vi "Pulse Generator Trigger.vi"() -> ()   [LabVIEW 2020]
uses:
  <vilib>/DAQmx/create/channels.llb/DAQmx Create Channel (CO-Pulse Generation-Time).vi
  <vilib>/DAQmx/configure/trigger.llb/DAQmx Start Trigger (Digital Edge).vi
  <resource>/objmgr/daqmx.rc
panel:
  in  "Output Terminal":tag
  in  "stop":bool
  in  "counter":tag
  in  "Trigger":tag
  in  "Low Time":dbl=0.0001
  in  "High Time":dbl=0.00025
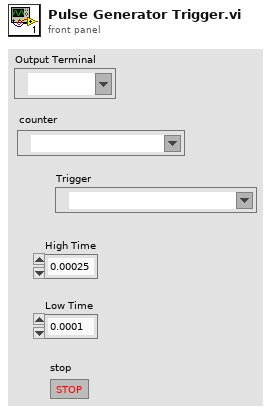
[diagram p1: front panel]
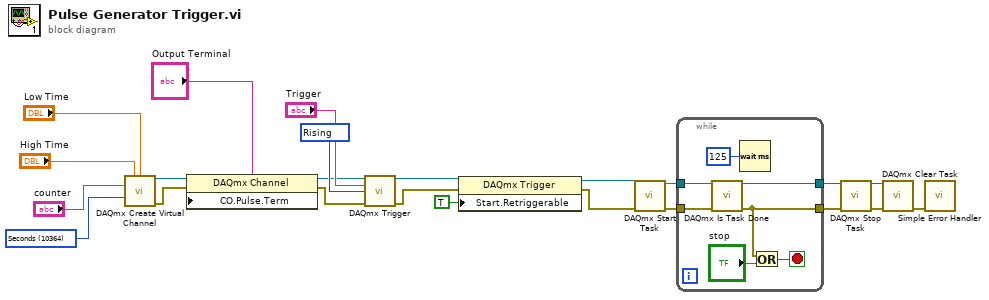
[diagram p0: block diagram]
diagram:
  w15 = 10364 items=["Seconds"=10364] ("units")
  w22 = 10280 items=["Rising"=10280, "Falling"=10171] ("edge")
  n1 = call-poly <vilib>:"DAQmx Create Virtual Channel.vi"("high time"="High Time", "low time"="Low Time", "counter"="counter", "units"=w15) -> ("task out"=w4:refnum<k21>, "error out"=w5:errorcluster)  [unwired: 10 in]
  n2 = property class="DAQmx Channel"(reference=w4, error in=w5, "CO.Pulse.Term"="Output Terminal") -> (reference out=w3:refnum<k21>, error out=w2:errorcluster)
  n3 = call-poly <vilib>:"DAQmx Trigger.vi"("task/channels in"=w3, "source"="Trigger", "edge"=w22, "error in"=w2) -> ("task out"=w10:refnum<k21>, "error out"=w9:errorcluster)  [unwired: 10 in]
  n4 = property class="DAQmx Trigger"(reference=w10, error in=w9, "Start.Retriggerable"=TRUE) -> (reference out=w8:refnum<k21>, error out=w7:errorcluster)
  n5 = call <vilib>:"DAQmx Start Task.vi"("task/channels in"=w8, "error in"=w7) -> ("task out"=w14:refnum<k21>, "error out"=w13:errorcluster)  [unwired: 12 in]
  n6 = while {
    tunnel: w14 -> [w30]
    tunnel: w13 -> [w29]
    tunnel: [w28] -> w12
    tunnel: [w27] -> w11
    stop <- w25 stop-if-true
    n7 = call <vilib>:"DAQmx Is Task Done.vi"("task/channels in"=w30, "error in"=w29) -> ("task out"=w28:refnum<k21>, "error out"=w27:errorcluster)  [unwired: 11 in, 1 out]
    n8 = Wait (ms)(milliseconds to wait=u32 125) -> ()  [unwired: 1 out]
    n9 = Or(x=w27, y="stop") -> (x .or. y?=w25:bool)
  }
  n10 = call <vilib>:"DAQmx Stop Task.vi"("task/channels in"=w12, "error in"=w11) -> ("task out"=w20:refnum<k21>, "error out"=w21:errorcluster)  [unwired: 12 in]
  n11 = call <vilib>:"DAQmx Clear Task.vi"("task in"=w20, "error in"=w21) -> ("error out"=w19:errorcluster)  [unwired: 13 in]
  n12 = call <vilib>:"Simple Error Handler.vi"("error in (no error)"=w19) -> ()  [unwired: 4 in, 5 out]
